vi "KB外环8通求最高点.vi"(7 "数值":i32, 11 "外环3D":dbl[][](array[numeric])) -> (0 "平均高度与最第高度差":dbl, 1 "最低高度":dbl, 2 "最大高度":dbl, 3 "平均高度":dbl, 4 "外环3D 2":dbl[][](array[numeric]))   [LabVIEW 2015]
uses:
  <vilib>/Math Plots/3D Math Plots/3D Surface/3D Surface XCtrl/3D Surface.xctl
  <vilib>/Math Plots/3D Math Plots/3D Surface/3D Surface Datatype/Public/Plot Helper (Matrix).vi
  <vilib>/Math Plots/3D Math Plots/3D Surface/3D Surface Datatype/3D Surface Datatype.lvclass
panel:
  out "大小 2":i32[](array[numeric])
  out "3D Surface 2":refnum<class "3D Plot Datatype.lvclass">[](xcontrol) caption="三维曲面"
  in  "内环3D":dbl[][](array[numeric])
  out "数组":dbl[](array[numeric])
  out "对角线第一 2":dbl[](graph)
  out "对角线第一":dbl[](graph)
  out "元素":dbl
  out "中间列波形":dbl[](graph)
  out "中间行波形":dbl[](graph)
  out "3D Surface":refnum<class "3D Plot Datatype.lvclass">[](xcontrol) caption="三维曲面"
  out "大小":i32[](array[numeric])
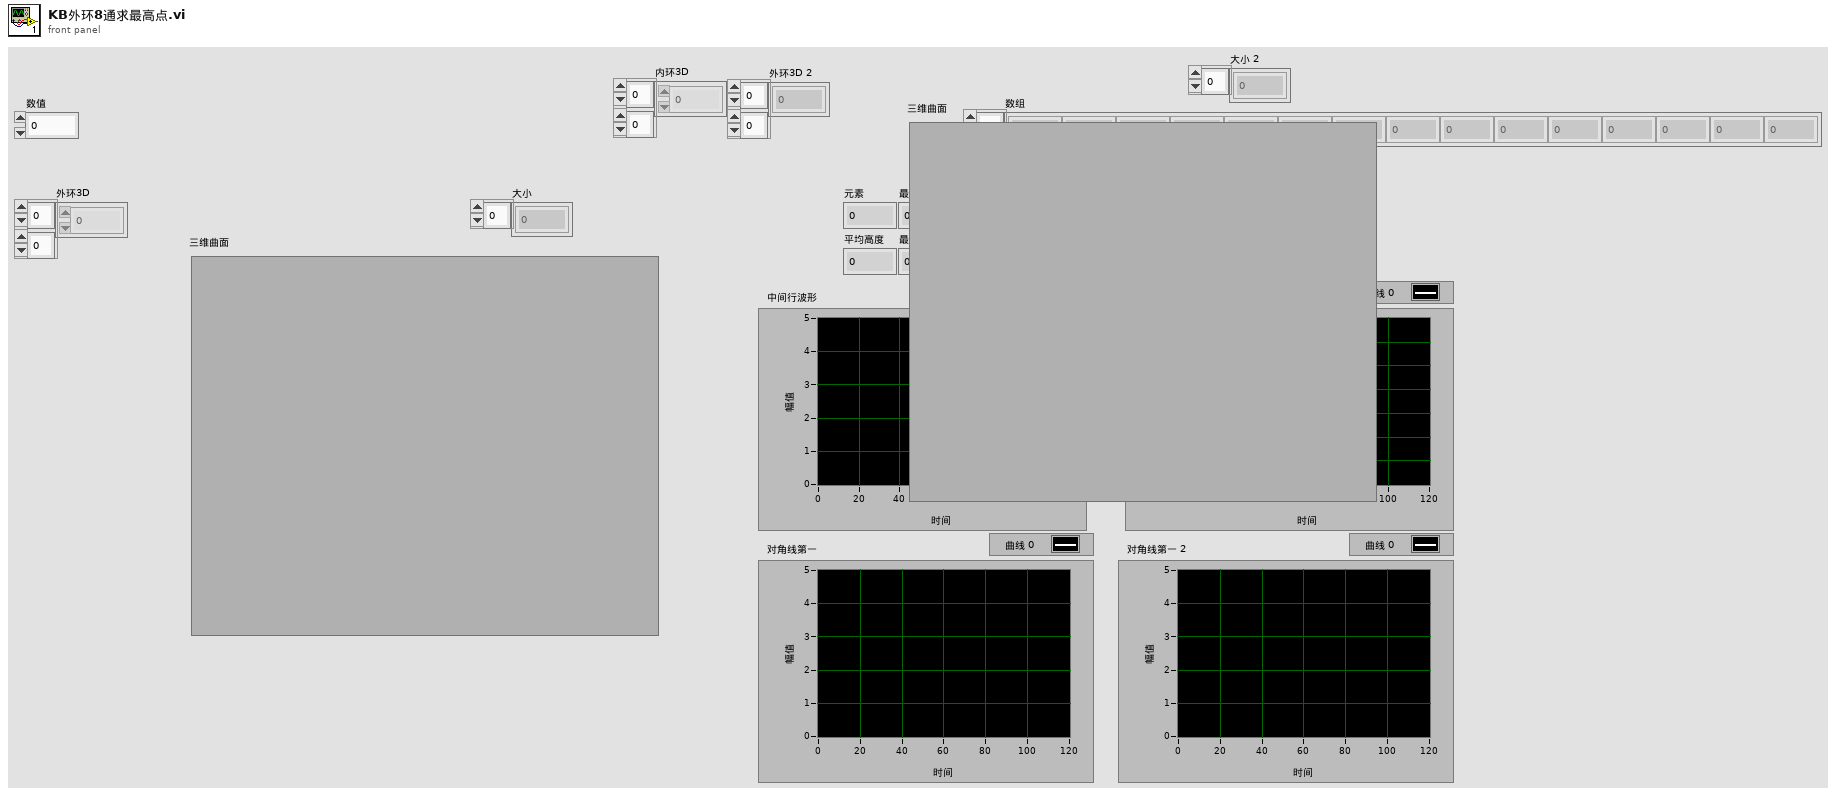
[diagram p1: front panel]
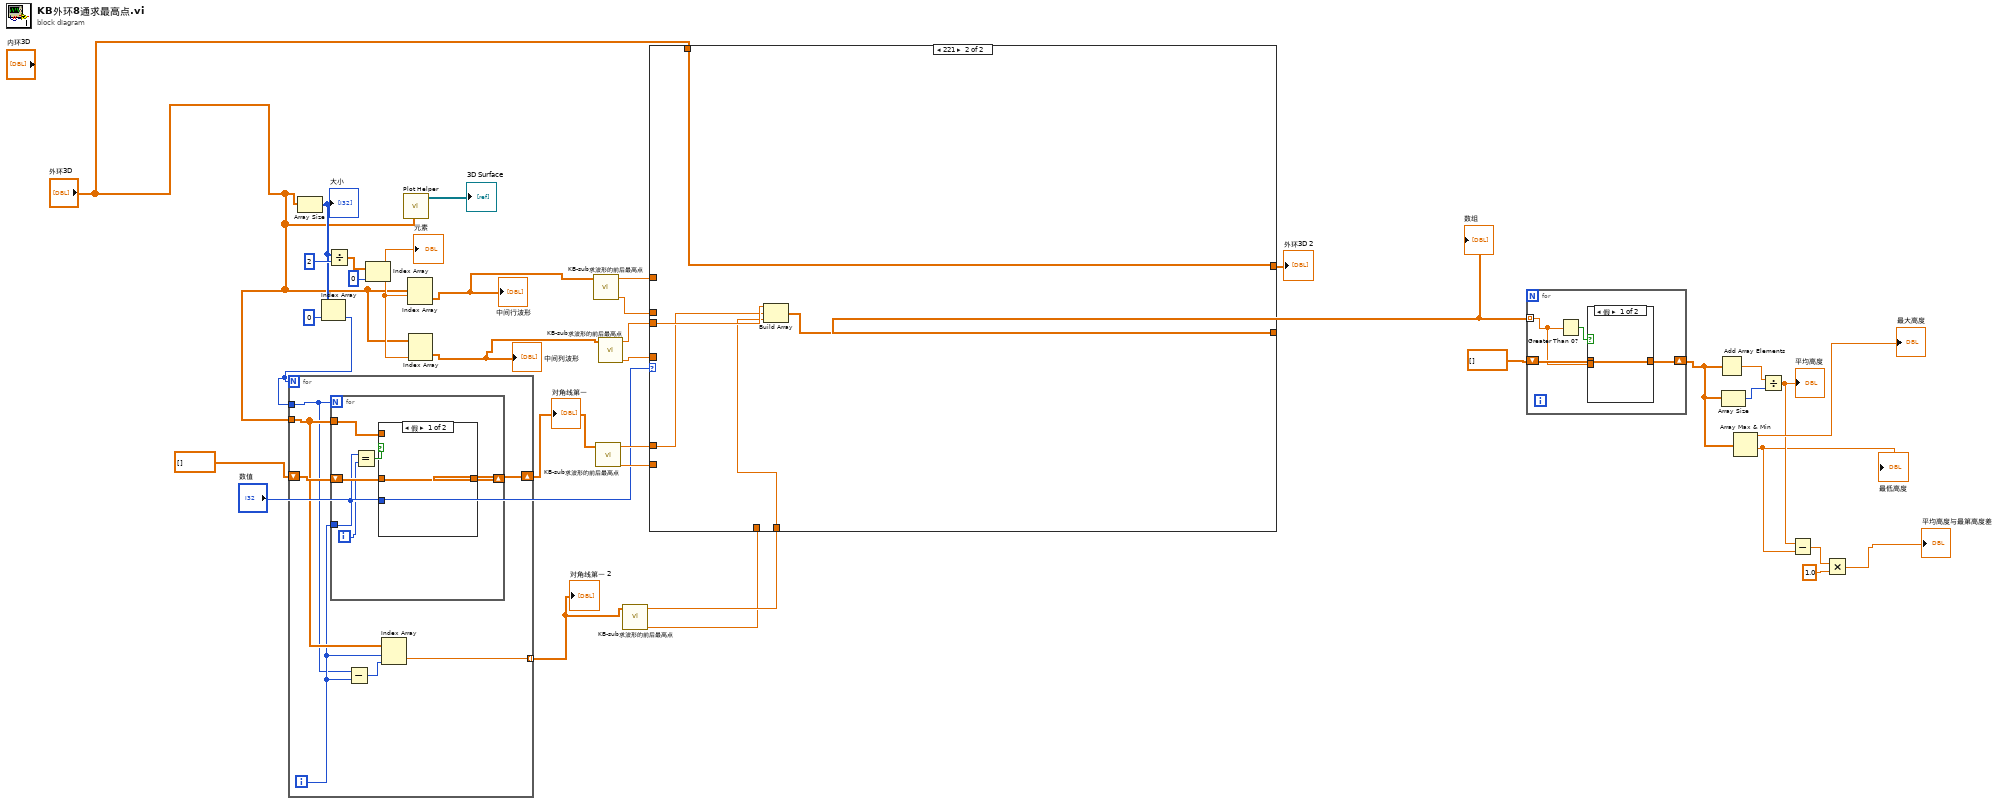
[diagram p0: block diagram]
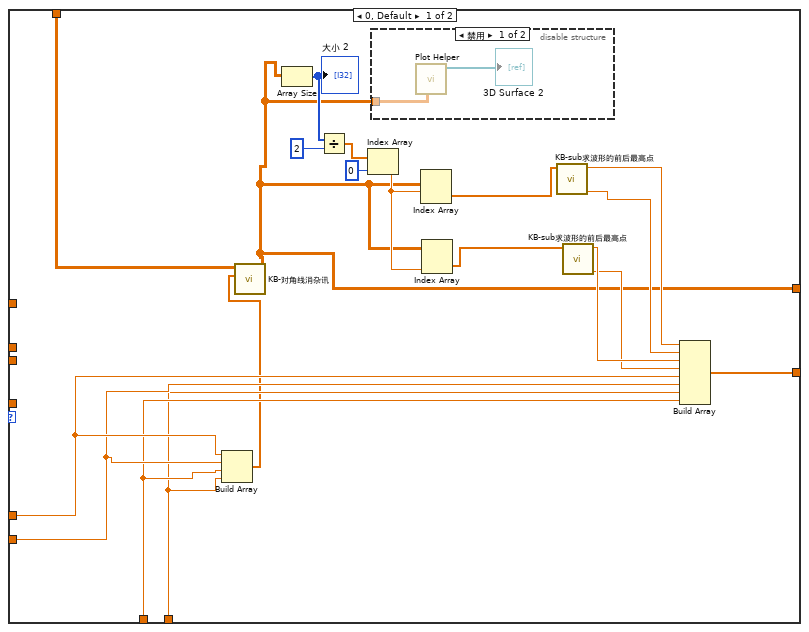
[diagram p2: hidden frame]
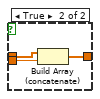
[diagram p4: hidden frame]
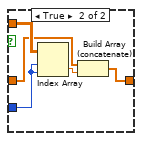
[diagram p5: hidden frame]
diagram:
  n1 = Array Size(array="外环3D") -> (size(s)=w30:i32[])
  "大小" <- w30
  n2 = Index Array(array=w30, index=0 ("索引")) -> (element=w28:i32)
  n3 = for {
    N: w28 -> [_]
    tunnel: "外环3D" -> [w40]
    tunnel: w28 -> [w38]
    shift-right: [w41] -> w24
    shift-left: dbl[] [] -> [w42]
    tunnel: [w36] -> w23 mode=indexing
    i -> [w39]
    n4 = for {
      N: w38 -> [_]
      tunnel: w40 -> [w46]
      shift-right: [w44] -> w41
      shift-left: w42 -> [w47]
      tunnel: w39 -> [w45]
      i -> [w43]
      n5 = Equal?(x=w45, y=w43) -> (x = y?=w48:bool)
      n6 = case shown="假" w48 {
        tunnel: w47 -> [w49 w51]
        tunnel: w46 -> [_ w54]
        tunnel: w45 -> [_ w53]
        tunnel: [w49 w50] -> w44
        frame False {
        }
        frame True {
          n7 = Index Array(array=w54, index (row)=w53, index (col)=w53) -> (element=w52:dbl)
          n8 = Build Array (concatenate)(w51, w52) -> (w50:dbl[])
        }
      }
    }
    n9 = Subtract(x=w38, y=w39) -> (x-y=w37:i32)
    n10 = Index Array(array=w40, index (row)=w39, index (col)=w37) -> (element=w36:dbl)
  }
  "对角线第一" <- w24
  "对角线第一 2" <- w23
  n11 = Divide(x=w30, y=2) -> (x/y=w33:dbl[])
  n12 = Index Array(array=w33, index=0 ("索引")) -> (element=w32:dbl)
  "元素" <- w32
  n13 = call-poly <vilib>:"Plot Helper.vi"("z matrix"="外环3D") -> ("3D Plot lvclass Array out"=→"3D Surface":refnum<class "3D Plot Datatype.lvclass">[])  [unwired: 5 in, 5 out]
  n14 = Index Array(array="外环3D", index (row)=w32) -> (element=w26:dbl[])  [unwired: 1 in]
  "中间行波形" <- w26
  n15 = Index Array(array="外环3D", index (col)=w32) -> (element=w25:dbl[])  [unwired: 1 in]
  "中间列波形" <- w25
  n16 = call "KB-sub求波形的前后最高点.vi"("中间行波形"=w26) -> ("后半部分高度平均值"=w21:dbl, "前半部分高度平均值"=w22:dbl)  [unwired: 9 in]
  n17 = call "KB-sub求波形的前后最高点.vi"("中间行波形"=w24) -> ("后半部分高度平均值"=w17:dbl, "前半部分高度平均值"=w18:dbl)  [unwired: 9 in]
  n18 = call "KB-sub求波形的前后最高点.vi"("中间行波形"=w25) -> ("后半部分高度平均值"=w19:dbl, "前半部分高度平均值"=w20:dbl)  [unwired: 9 in]
  n19 = call "KB-sub求波形的前后最高点.vi"("中间行波形"=w23) -> ("后半部分高度平均值"=w15:dbl, "前半部分高度平均值"=w16:dbl)  [unwired: 9 in]
  n20 = case shown="221" "数值" {
    tunnel: w22 -> [_ _]
    tunnel: w21 -> [_ _]
    tunnel: w20 -> [_ w80]
    tunnel: w19 -> [_ _]
    tunnel: w18 -> [w71 w79]
    tunnel: w17 -> [w70 _]
    tunnel: w16 -> [w68 w78]
    tunnel: w15 -> [w69 _]
    tunnel: [w73 w77] -> w13
    tunnel: "外环3D" -> [w72 w76]
    tunnel: [w55 w76] -> w1
    frame 0, Default {
      n21 = Build Array(w71, w70, w69, w68) -> (w67:dbl[])
      n22 = call "KB-对角线消杂讯.vi"("对角线高度值"=w67, "外环3D"=w72) -> ("消杂讯数据"=w55:dbl[][])  [unwired: 9 in]
      n23 = Array Size(array=w55) -> (size(s)=w65:i32[])
      "大小 2" <- w65
      n24 = Divide(x=w65, y=2) -> (x/y=w63:dbl[])
      n25 = Index Array(array=w63, index=0 ("索引")) -> (element=w61:dbl)
      n26 = disable-structure shown="禁用" {
        disable-tunnel: w55 -> [w74 _]
        frame Disabled {
          n27 = call-poly <vilib>:"Plot Helper.vi"("z matrix"=w74) -> ("3D Plot lvclass Array out"=→"3D Surface 2":refnum<class "3D Plot Datatype.lvclass">[])  [unwired: 5 in, 5 out]
        }
        frame Enabled {
        }
      }
      n28 = Index Array(array=w55, index (row)=w61) -> (element=w66:dbl[])  [unwired: 1 in]
      n29 = Index Array(array=w55, index (col)=w61) -> (element=w60:dbl[])  [unwired: 1 in]
      n30 = call "KB-sub求波形的前后最高点.vi"("中间行波形"=w66) -> ("后半部分高度平均值"=w58:dbl, "前半部分高度平均值"=w59:dbl)  [unwired: 9 in]
      n31 = call "KB-sub求波形的前后最高点.vi"("中间行波形"=w60) -> ("后半部分高度平均值"=w56:dbl, "前半部分高度平均值"=w57:dbl)  [unwired: 9 in]
      n32 = Build Array(w59, w58, w57, w56, w71, w70, w68, w69) -> (w73:dbl[])
    }
    frame 221 {
      n33 = Build Array(w80, w79, w78) -> (w77:dbl[])
    }
  }
  "数组" <- w13
  "外环3D 2" <- w1
  n34 = for {
    tunnel: w13 -> [w82] mode=indexing
    shift-right: [w81] -> w10
    shift-left: dbl[] [] -> [w83]
    n35 = Greater Than 0?(x=w82) -> (x > 0?=w84:bool)
    n36 = case shown="假" w84 {
      tunnel: w83 -> [w85 w88]
      tunnel: w82 -> [_ w87]
      tunnel: [w85 w86] -> w81
      frame False {
      }
      frame True {
        n37 = Build Array (concatenate)(w88, w87) -> (w86:dbl[])
      }
    }
  }
  n38 = Add Array Elements(numeric array=w10) -> (sum=w12:dbl)
  n39 = Array Size(array=w10) -> (size(s)=w11:i32)
  n40 = Array Max & Min(array=w10) -> (max value=→"最大高度":dbl, min value=w7:dbl)  [unwired: 2 out]
  "最低高度" <- w7
  n41 = Divide(x=w12, y=w11) -> (x/y=w8:dbl)
  "平均高度" <- w8
  n42 = Subtract(x=w8, y=w7) -> (x-y=w4:dbl)
  n43 = Multiply(x=w4, y=1.0) -> (x*y=→"平均高度与最第高度差":dbl)
